vi "Create_Simplified.vi"(4 "request headers":cluster{"header":string, "value":string}[](array[cluster]), 5 "input file":path, 6 "ContentType":T1, 7 "Method [GET]":T2, 8 "error in (no error)":errorcluster, 10 "buffer":string, 11 "Address":string) -> (0 "error out":errorcluster, 2 "RequestHeaders":refnum<class "HttpHeaders_Request.lvclass">, 3 "HttpRequestMessage out":refnum<class "HttpRequestMessage.lvclass">)   [LabVIEW 2018, in "LabVIEWHTTPClient_NET.lvlib" / "HttpRequestMessage.lvclass"]
uses:
  HttpRequestMessage.lvclass
  Types/method_enum.ctl
  Types/ContentType.ctl
  HttpHeaders_Request/HttpHeaders_Request.lvclass
  C:/Viviota/Projects/R&D/LabVIEW_HTTP_REST_NET/HTTPHeaders_NET/HttpHeaders_NET.lvclass
  HttpContent_Stream/HttpContent_Stream.lvclass
  C:/Viviota/Projects/R&D/LabVIEW_HTTP_REST_NET/HttpContent/HttpContent.lvclass
  HttpContent_ByteArray/HttpContent_ByteArray.lvclass
  HttpHeaders_content/HttpHeaders_Content.lvclass
  HttpContent/HttpContent.lvclass
  LabVIEWHTTPClient_NET/LabVIEWHTTPClient_NET.lvlib
  HTTPHeaders_NET/HttpHeaders_NET.lvclass
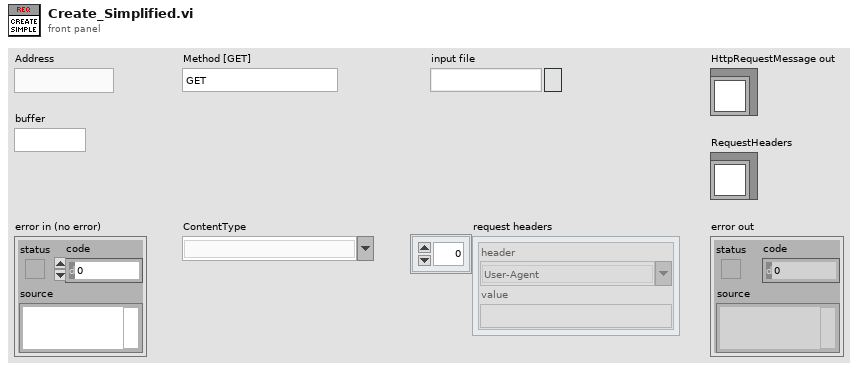
[diagram p1: front panel]
types:
  T1 = typedef "LabVIEWHTTPClient_NET.lvlib/ContentType.ctl" = string
  T2 = typedef "LabVIEWHTTPClient_NET.lvlib/method_enum.ctl" = enum16{"GET", "PUT", "POST", "DELETE", "HEAD", "TRACE", "SEND"}
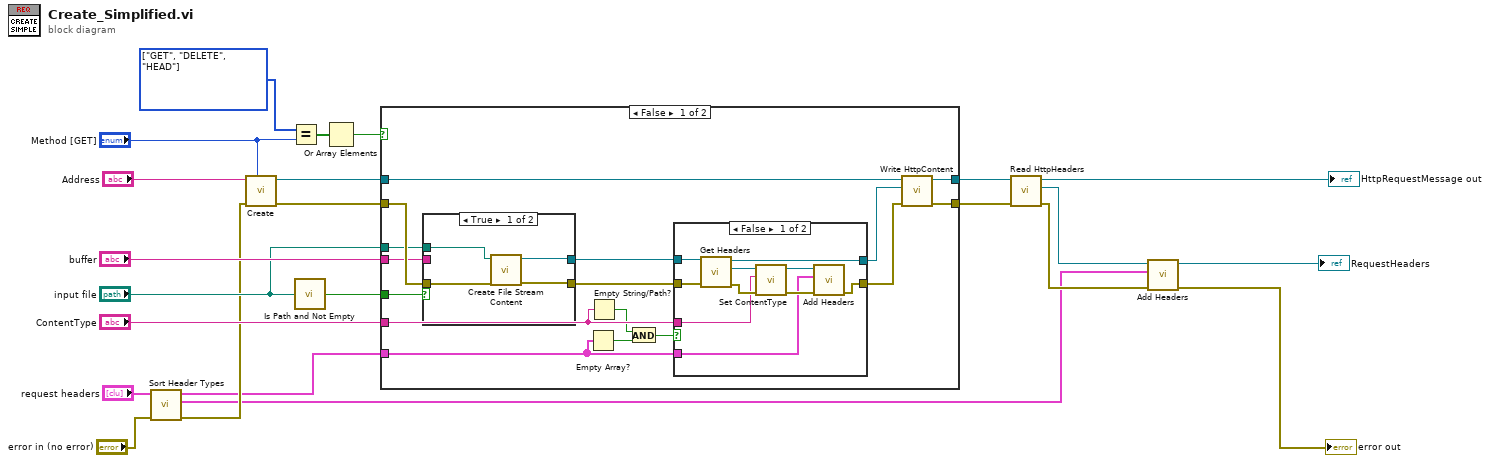
[diagram p0: block diagram]
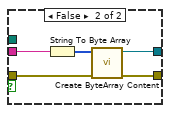
[diagram p3: hidden frame]
diagram:
  w10 = T2[] [enum."GET", enum."DELETE", enum."HEAD"] items=["GET", "PUT", "POST", "DELETE", "HEAD", "TRACE", "SEND"]
  n1 = call "Sort Header Types.vi"("error in (no error)"="error in (no error)", "request headers"="request headers") -> ("error out"=w7:errorcluster, "Request Headers"=w2:cluster{"header":string, "value":string}[], "Content-Headers"=w1:cluster{"header":string, "value":string}[])  [unwired: 7 in]
  n2 = call "Create.vi"("Method [GET]"="Method [GET]", "error in (no error)"=w7, "Address"="Address") -> ("error out"=w21:errorcluster, "HttpRequestMessage out"=w22:refnum<class "HttpRequestMessage.lvclass">)  [unwired: 7 in]
  n3 = Equal?(x=w10, y="Method [GET]") -> (x = y?=w9:bool[])
  n4 = call <vilib>:"Is Path and Not Empty.vi"("path"="input file") -> ("Is Path and Not Empty?"=w19:bool)  [unwired: 4 in]
  n5 = Or Array Elements(Boolean array=w9) -> (logical OR=w8:bool)
  n6 = case shown="False" w8 {
    tunnel: w22 -> [w39 w61]
    tunnel: w21 -> [w38 w62]
    tunnel: "buffer" -> [w37 _]
    tunnel: w19 -> [w36 _]
    tunnel: "input file" -> [w35 _]
    tunnel: [w34 w62] -> w17
    tunnel: [w33 w61] -> w16
    tunnel: "ContentType" -> [w27 _]
    tunnel: w1 -> [w28 _]
    frame False {
      n7 = case shown="True" w36 {
        tunnel: [w53 w59] -> w32
        tunnel: [w54 w60] -> w31
        tunnel: w38 -> [w55 w58]
        tunnel: w37 -> [_ w57]
        tunnel: w35 -> [w52 _]
        frame True {
          n8 = call "Create File Stream Content.vi"("error in (no error)"=w55, "File"=w52) -> ("error out"=w54:errorcluster, "HttpContent_Stream out"=w53:refnum<class "HttpContent_Stream.lvclass">)  [unwired: 8 in]
        }
        frame False {
          n9 = String To Byte Array(string=w57) -> (unsigned byte array=w56:u8[])
          n10 = call "Create ByteArray Content.vi"("error in (no error)"=w58, "content"=w56) -> ("error out"=w60:errorcluster, "HttpContent_String out"=w59:refnum<class "HttpContent_ByteArray.lvclass">)  [unwired: 8 in]
        }
      }
      n11 = Empty Array?(array=w28) -> (empty?=w26:bool)
      n12 = Empty String/Path?(string/path=w27) -> (empty?=w25:bool)
      n13 = And(x=w25, y=w26) -> (x .and. y?=w24:bool)
      n14 = case shown="False" w24 {
        tunnel: w32 -> [w49 w50]
        tunnel: w31 -> [w48 w51]
        tunnel: [w45 w50] -> w30
        tunnel: [w42 w51] -> w29
        tunnel: w27 -> [w44 _]
        tunnel: w28 -> [w40 _]
        frame False {
          n15 = call "Get Headers.vi"("error in (no error)"=w48, "HttpContent in"=w49) -> ("error out"=w46:errorcluster, "HTTPHeaders"=w47:refnum<class "HttpHeaders_Content.lvclass">, "HttpContent out"=w45:refnum<class "HttpContent.lvclass">)  [unwired: 7 in]
          n16 = call "Set ContentType.vi"("error in (no error)"=w46, "ContentType"=w44, "HttpHeaders_Content in"=w47) -> ("error out"=w43:errorcluster, "HttpHeaders_Content out"=w41:refnum<class "HttpHeaders_Content.lvclass">)  [unwired: 7 in]
          n17 = call "Add Headers.vi"("error in (no error)"=w43, "headers"=w40, "HttpHeaders_NET in"=w41) -> ("error out"=w42:errorcluster)  [unwired: 7 in, 1 out]
        }
        frame True {
        }
      }
      n18 = call "Write HttpContent.vi"("error in (no error)"=w29, "HttpContent"=w30, "HttpRequestMessage in"=w39) -> ("error out"=w34:errorcluster, "HttpRequestMessage out"=w33:refnum<class "HttpRequestMessage.lvclass">)  [unwired: 7 in]
    }
    frame True {
    }
  }
  n19 = call "Read HttpHeaders.vi"("error in (no error)"=w17, "HttpRequestMessage in"=w16) -> ("error out"=w3:errorcluster, "HttpHeaders"=w6:refnum<class "HttpHeaders_Request.lvclass">, "HttpRequestMessage out"=→"HttpRequestMessage out":refnum<class "HttpRequestMessage.lvclass">)  [unwired: 7 in]
  n20 = call "Add Headers.vi"("error in (no error)"=w3, "headers"=w2, "HttpHeaders_NET in"=w6) -> ("error out"=→"error out":errorcluster, "HttpHeaders_NET out"=→"RequestHeaders":refnum<class "HttpHeaders_Request.lvclass">)  [unwired: 7 in]
